vi "test - FGV Simple Register and Unregister.vi"(8 "error in (no error)":errorcluster, 11 "TestCase in":refnum<class "testcase-Broadcast Registry.lvclass">) -> (0 "error out":errorcluster, 3 "TestCase out":refnum<class "testcase-Broadcast Registry.lvclass">)   [LabVIEW 2017, in "testcase-Broadcast Registry.lvclass"]
uses:
  testcase-Broadcast Registry.lvclass
  <vilib>/addons/_JKI Toolkits/VI Tester/TestCase.llb/TestCase.lvclass
  C:/Program Files (x86)/National Instruments/LabVIEW 2017/vi.lib/addons/_JKI Toolkits/VI Tester/TestCase.llb/TestCase.lvclass
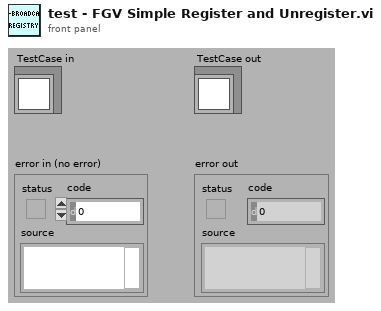
[diagram p1: front panel]
types:
  T1 = cluster{"response message":string[], "response message":string[]}
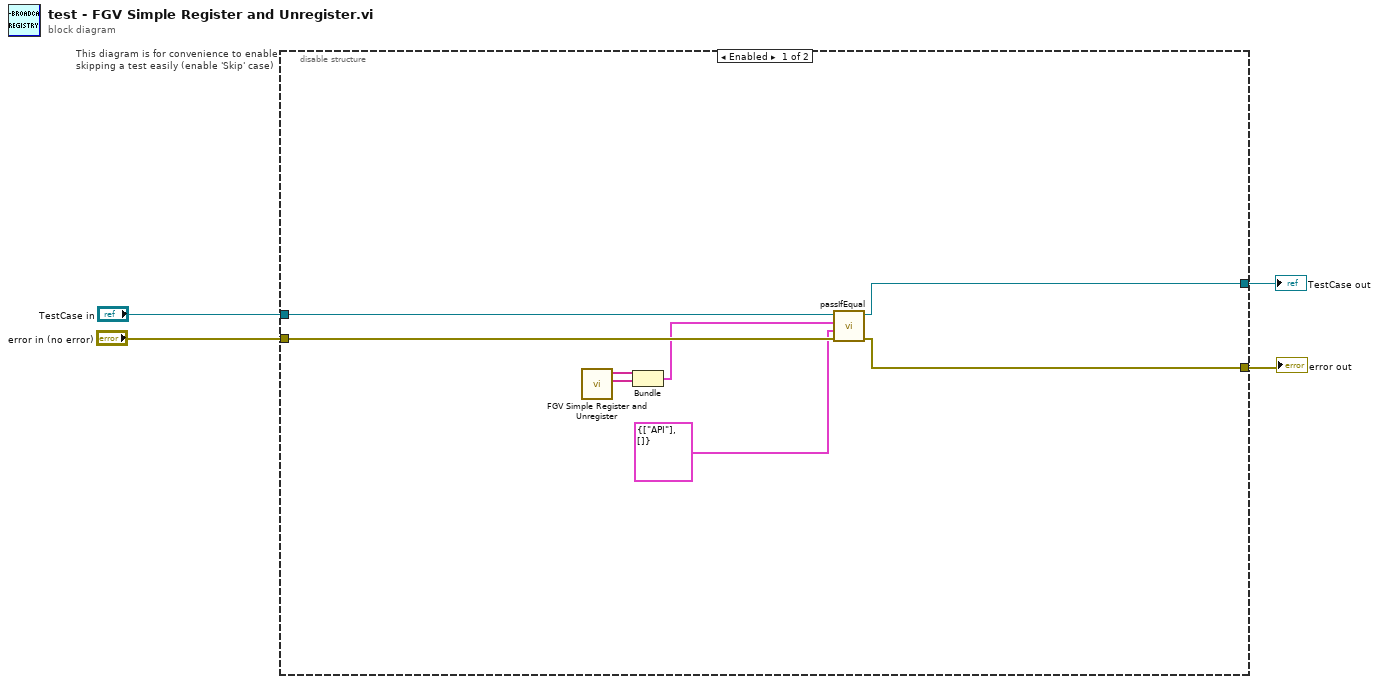
[diagram p0: block diagram]
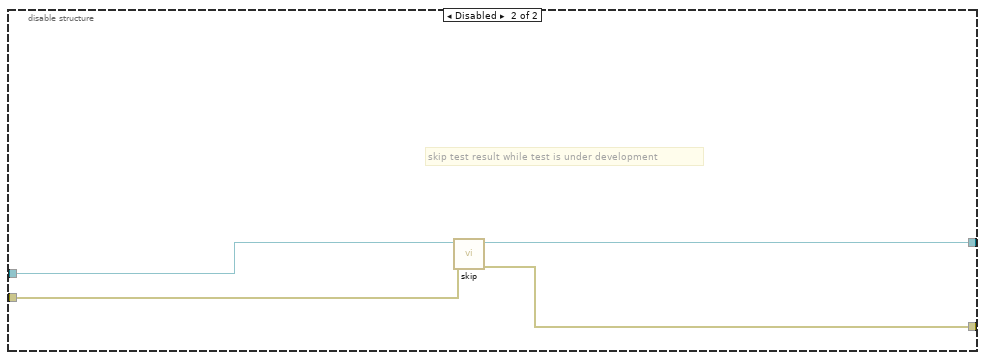
[diagram p2: hidden frame]
diagram:
  n1 = disable-structure "This diagram is for convenience to enable skipping a test easily (enable 'Skip' case)" shown="Enabled" {
    disable-tunnel: "TestCase in" -> [w12 w16]
    disable-tunnel: [w9 w14] -> w1
    disable-tunnel: [w10 w15] -> w3
    disable-tunnel: "error in (no error)" -> [w11 w13]
    frame Enabled {
      n2 = call "FGV Simple Register and Unregister.vi"() -> (2:"response message"=w7:string[], 3:"response message"=w8:string[])  [unwired: 10 in]
      n3 = Bundle("response message"=w8, "response message"=w7) -> (w5:T1)  [unwired: 1 in]
      n4 = call-dynamic "passIfEqual.vi"("error in (no error)"=w11, "y"=T1 {"response message"=["API"], "response message"=[]} ("output cluster"), "x"=w5, "TestCase in"=w12) -> ("error out"=w10:errorcluster, "TestCase out"=w9:refnum<class "testcase-Broadcast Registry.lvclass">)  [unwired: 6 in]
    }
    frame Disabled {
      # "skip test result while test is under development"
      n5 = call <vilib>:"skip.vi"("error in (no error)"=w13, "TestCase in"=w16) -> ("error out"=w15:errorcluster, "TestCase out"=w14:refnum<class "testcase-Broadcast Registry.lvclass">)  [unwired: 8 in]
    }
  }
  "error out" <- w3
  "TestCase out" <- w1
